vi "PLL_PID.vi"() -> ()   [LabVIEW 2019]
doc: "Please ensure that at least one period is generated or else the measurement VIs do not work properly."
uses:
  <vilib>/measure/matone.llb/Extract Single Tone Information 1 Chan.vi
  <vilib>/addons/control/pid/pid.llb/PID (DBL).vi
  <vilib>/measure/NI_MABase.lvlib
  <vilib>/Analysis/NI_AALPro.lvlib
  <vilib>/measure/NI_MAPro.lvlib
  <vilib>/addons/control/pid/NI_PID_pid.lvlib
panel:
  in  "PID_Phase":T1={"proportional gain (Kc)"=0.1, "integral time (Ti, min)"=0.0008, "derivative time (Td, min)"=0.0} {"derivative time (Td, min)" format="%.3f"; "integral time (Ti, min)" items=["Take a Coffee"=0.1, "Yawning"=0.01, "Take a Deep Breath"=0.001, "Normal"=0.0008, "A Little Bit Fast"=0.0001, "Fast"=1e-05, "Too Fast"=1e-06]; "proportional gain (Kc)" format="%.3f"}
  out "Current Frequency [Hz]":dbl=10.000000000000004 format="%.2f"
  in  "PID_Frequency":T1={"proportional gain (Kc)"=0.9, "integral time (Ti, min)"=0.0008, "derivative time (Td, min)"=0.0} {"derivative time (Td, min)" format="%.3f"; "integral time (Ti, min)" items=["Take a Coffee"=0.1, "Yawning"=0.01, "Take a Deep Breath"=0.001, "Normal"=0.0008, "A Little Bit Fast"=0.0001, "Fast"=1e-05, "Too Fast"=1e-06]; "proportional gain (Kc)" format="%.3f"}
  out "Waveform Graph":waveform(dbl)[](graph)=[{"t0"=timestamp(0 s since 1904-01-01), "dt"=0.001, "Y"=array[1000 elements]}, {"t0"=timestamp(0 s since 1904-01-01), "dt"=0.001, "Y"=array[1000 elements]}]
  in  "stop":bool
  in  "sampling info":cluster{"Fs":dbl, "#s":dbl}={"Fs"=1000.0, "#s"=1000.0} {"Fs" format="%.2p"}
  in  "Desired Frequency [Hz]":dbl=10.0 format="%_6f"
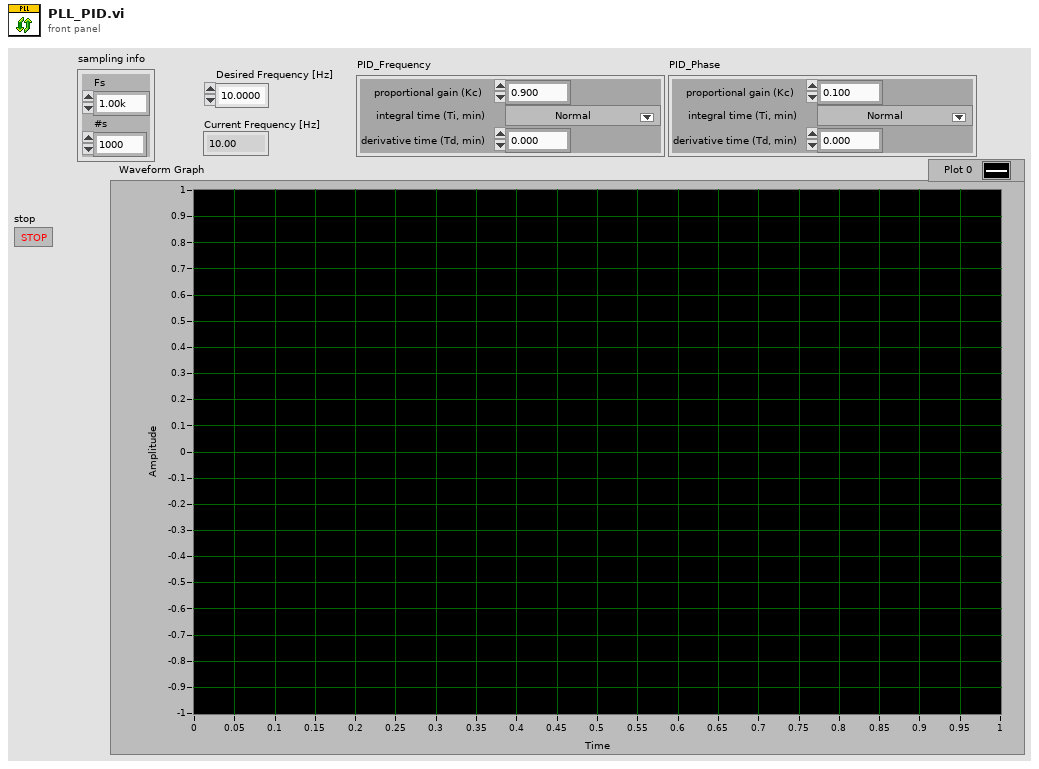
[diagram p1: front panel]
types:
  T1 = cluster{"proportional gain (Kc)":dbl, "integral time (Ti, min)":dbl, "derivative time (Td, min)":dbl}
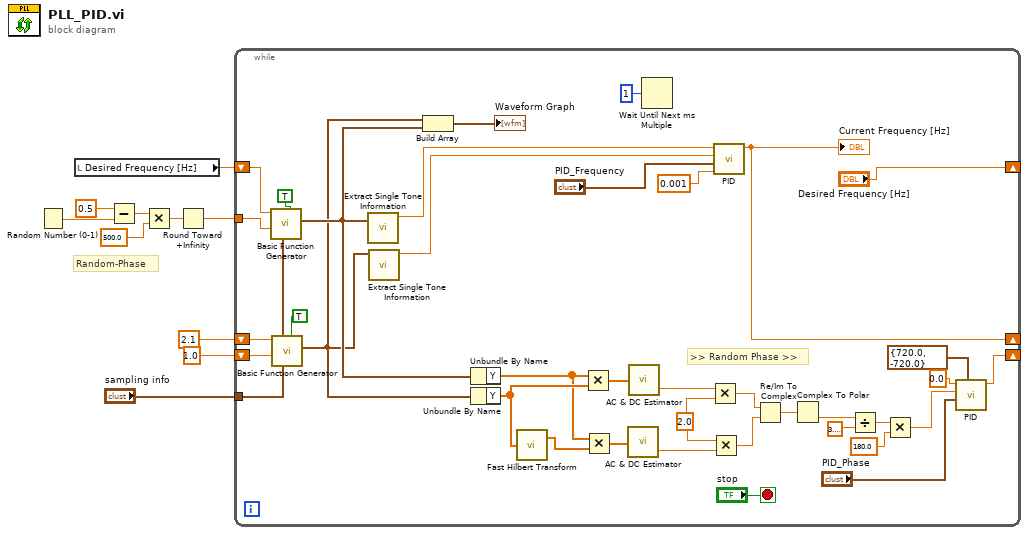
[diagram p0: block diagram]
diagram:
  # "Random-Phase"
  n1 = Random Number (0-1)() -> (number: 0 to 1=w8:dbl)
  n2 = local read "Desired Frequency [Hz]"() -> (w1:dbl)
  n3 = Subtract(x=0.5, y=w8) -> (x-y=w2:dbl)
  n4 = Multiply(x=w2, y=500.0) -> (x*y=w5:dbl)
  n5 = Round Toward +Infinity(x=w5) -> (ceil(x): smallest int >= x=w4:dbl)
  n6 = while {
    tunnel: "sampling info" -> [w48]
    shift-right: [w13] -> _
    shift-left: 1.0 -> [w29]
    tunnel: w4 -> [w16]
    shift-right: [w18] -> _
    shift-left: 2.1 ("f") -> [w43]
    shift-right: ["Desired Frequency [Hz]"] -> _
    shift-left: w1 -> [w22]
    stop <- "stop" stop-if-true
    w27 = 2.0 ("x")
    # ">> Random Phase >>"
    n7 = call <vilib>:"Basic Function Generator.vi"("reset signal"=TRUE, "sampling info"=w48, "phase"=w16, "frequency"=w22) -> ("signal out"=w26:waveform(dbl))  [unwired: 5 in, 2 out]
    n8 = call <vilib>:"Basic Function Generator.vi"("reset signal"=TRUE, "sampling info"=w48, "phase"=w29, "frequency"=w43) -> ("signal out"=w25:waveform(dbl))  [unwired: 5 in, 2 out]
    n9 = call-poly <vilib>:"Extract Single Tone Information.vi"("time signal in"=w26) -> ("detected frequency"=w21:dbl)  [unwired: 5 in, 5 out]
    n10 = call-poly <vilib>:"Extract Single Tone Information.vi"("time signal in"=w25) -> ("detected frequency"=w20:dbl)  [unwired: 5 in, 5 out]
    n11 = Build Array(w25, w26) -> (→"Waveform Graph":waveform(dbl)[])
    n12 = Unbundle By Name(w26) -> ("Y"=w40:dbl[])
    n13 = Unbundle By Name(w25) -> ("Y"=w42:dbl[])
    n14 = call <vilib>:"Fast Hilbert Transform.vi"("X"=w42) -> ("Hilbert{X}"=w41:dbl[])  [unwired: 1 out]
    n15 = Multiply(x=w40, y=w42) -> (x*y=w39:dbl[])
    n16 = Multiply(x=w40, y=w41) -> (x*y=w38:dbl[])
    n17 = call <vilib>:"AC & DC Estimator.vi"("Signal (V)"=w38) -> ("DC estimate (V)"=w37:dbl)  [unwired: 1 out]
    n18 = call <vilib>:"AC & DC Estimator.vi"("Signal (V)"=w39) -> ("DC estimate (V)"=w28:dbl)  [unwired: 1 out]
    n19 = Wait Until Next ms Multiple(millisecond multiple=u32 1) -> ()  [unwired: 1 out]
    n20 = Multiply(x=w28, y=w27) -> (x*y=w31:dbl)
    n21 = Multiply(x=w27, y=w37) -> (x*y=w30:dbl)
    n22 = call-poly <vilib>:"PID.vi"("dt (s)"=0.001, "PID gains"="PID_Frequency", "process variable"=w20, "setpoint"=w21) -> ("output"=w18:dbl)  [unwired: 6 in, 1 out]
    "Current Frequency [Hz]" <- w18
    n23 = Re/Im To Complex(1:w30, 2:w31) -> (0:w32:cdb)
    n24 = Complex To Polar(r * e^(i*theta)=w32) -> (theta=w33:dbl)  [unwired: 1 out]
    n25 = Divide(x=w33, y=3.141592653589793) -> (x/y=w35:dbl)
    n26 = Multiply(x=w35, y=180.0) -> (x*y=w14:dbl)
    n27 = call-poly <vilib>:"PID.vi"("output range"=cluster{"output high":dbl, "output low":dbl} {"output high"=720.0, "output low"=-720.0}, "PID gains"="PID_Phase", "process variable"=w14, "setpoint"=0.0) -> ("output"=w13:dbl)  [unwired: 6 in, 1 out]
  }
